vi "Fsweep_SR8XX_2.vi"() -> ()   [LabVIEW 2024]
panel:
  out "Array":dbl[](array[numeric])=[40.99999999999999, 41.74838432440391, 42.51042911458864, 43.28638371880915, 44.07650203674304, 44.88104260256878, 45.70026866956066, 46.53444829622764, 47.38385443402472, 48.248765016665224, 49.129463051063276, 50.02623670993638, 50.93937942609823, 51.86918998847271, 52.815972639860554, 53.78003717649025, 54.761699049386465, 55.76127946758855, 56.779105503253135, 57.81551019867534, 58.87083267526322, 59.94541824450158, 61.039618520941126, 62.153791537250044, 63.28830186136581, 64.44352071578506, 65.61982609903121, 66.81760290933916, 68.03724307059753, 69.27914566059006, 70.5437170415774, 71.83137099326281, 73.14252884818475, 74.47761962958087, 75.83708019176856, 77.22135536308764, 78.6308980914525, 80.0661695925609, 81.5276395008081, 83.01578602295587, 84.53109609460586, 86.07406553952985, 87.64519923190788, 89.24501126152778, 90.87402510200042, 92.53277378204491, 94.22180005990091, 95.94165660092408, 97.6929061584234, 99.47612175779966, 101.29188688404435, 103.14079567266168, 105.02345310407557, 106.94047520158428, 108.89248923292998, 110.88013391554568, 112.90405962555053, 114.96492861055856, 117.06341520637208, 119.20020605763142, 121.37600034249118, 123.59151000139757, 125.84745997004288, 128.14458841657034, 130.48364698311073, 132.8654010317256, 135.2906298948422, 137.76012713025767, 140.27470078079847, 142.8351736387203, 145.44238351493328, 148.09718351314098, 150.80044230898505, 153.55304443428304, 156.35589056645665, 159.2098978232407, 162.11600006277385, 165.07514818916525, 168.08831046363892, 171.15647282135896, 174.28063919403635, 177.46183183842433, 180.70109167081173, 183.9994786076192, 187.35807191221528, 190.77797054806013, 194.26029353829807, 197.80618033191195, 201.41679117656102, 205.09330749822615, 208.83693228778293, 212.64889049463108, 216.53042942751085, 220.4828191626326, 224.50735295925946, 228.60534768287218, 232.7781442360615, 237.02710799728362, 241.353629267624, 245.75912372571858, 250.2450328909765, 254.81282459525804, 259.46399346316485, 264.2000614010933, 269.02257809521853, 273.93312151856446, 278.93329844733324, 284.02474498665686, 289.20912710594536, 294.4881411840093, 299.8635145641304, 305.3370061192634, 310.91040682755784, 316.58554035838205, 322.36426366904453, 328.2484676124084, 334.24007755559677, 340.341054009991, 346.55339327272696, 352.87912807990466, 359.3203282717176, 365.8791014697228, 372.55759376647694, 379.35799042775693, 386.28251660759867, 393.33343807638926, 400.5130619622492, 407.823737505946, 415.26785682958644, 422.847855719344, 430.5662144224702, 438.42545845885314, 446.4281594473945, 454.5769359474659, 462.8744543157258, 471.3234295785769, 479.92662632054976, 488.6868595889001, 497.60699581471715, 506.68995375085, 515.9387054269498, 525.356277121944, 534.9457503542673, 544.7102628901607, 554.6530097703788, 564.7772443556371, 575.086279391144, 585.5834880905614, 596.2723052397499, 607.1562283206671, 618.2388186557745, 629.5237025733345, 641.0145725939827, 652.7151886389541, 664.6293792603626, 676.7610428939417, 689.1141491346505, 701.6927400355609, 714.5009314304542, 727.5429142805647, 740.8229560458996, 754.3454020815899, 768.1146770597366, 782.1352864172023, 796.411817829832, 810.9489427135836, 825.7514177530663, 840.8240864579619, 856.1718807478732, 871.7998225660953, 887.7130255228415, 903.9166965684622, 920.416137697213, 937.2167476821156, 954.3240238414847, 971.7435638377035, 989.4810675088389, 1007.5423387336702, 1025.9332873307803, 1044.659930992305, 1063.7283972529765, 1083.1449254951083, 1102.9158689901853, 1123.0476969777121, 1143.5469967820063, 1164.4204759676343, 1185.6749645341988, 1207.3174171511644, 1229.3549154334992, 1251.7946702588479, 1274.644024126997, 1297.9104535624053, 1321.6015715606015, 1345.725130079225, 1370.2890225745357, 1395.3012865842295, 1420.770106357407, 1446.7038155325192, 1473.1108998642226, 1500.0000000000005]
  in  "data acq time (s)":dbl=2.0
  in  "restart":bool
  in  "stop":bool
  in  "coupled device":enum16{"SRS 8XXX", "Keithley 6221"}(ring)
  in  "base delay (ms)":dbl=2000.0
  in  "test mode":bool
  out "done":u32
  out "delays (ms)":dbl[](array[numeric])=[4439.024390243903, 4395.302276201986, 4352.363927695151, 4310.195294890093, 4268.7825798117565, 4228.112231828511, 4188.170943218251, 4148.945644813986, 4110.423501727488, 4072.5919091495875, 4035.438488225769, 3998.9510820056885, 3963.1177514653054, 3927.9267716003233, 3893.3666275896503, 3859.4260110276505, 3826.093816223921, 3793.359136569407, 3761.2112609676556, 3729.639670330042, 3698.634034133829, 3668.184207041918, 3638.2802255832016, 3608.9123048924207, 3580.0708355084616, 3551.7463802300545, 3523.9296710278295, 3496.6116060117283, 3469.7832464527837, 3443.435813858278, 3417.5606870993415, 3392.1493995900364, 3367.1936365170095, 3342.685232118807, 3318.6161670139577, 3294.978565576961, 3271.7646933613037, 3248.966954568677, 3226.577889563561, 3204.590172432356, 3182.996608586284, 3161.790132407242, 3140.96380493587, 3120.5108116010574, 3100.4244599901485, 3080.698177659125, 3061.3255099820385, 3042.300118038996, 3023.615776542007, 3005.2663717980067, 2987.2458997084013, 2969.5484638044713, 2952.168273317985, 2935.099641286413, 2918.3369826920916, 2901.8748126347614, 2885.707744536847, 2869.8304883809224, 2854.2378489787707, 2838.9247242714628, 2823.8861036599187, 2809.117066365394, 2794.612779819349, 2780.3684980821945, 2766.379560290368, 2752.6413891312604, 2739.149489345473, 2725.899446255926, 2712.8869243233385, 2700.1076657275935, 2687.557488974543, 2675.232287527783, 2663.128028464952, 2651.2407511581287, 2639.566565977868, 2628.101653020485, 2616.8422608581413, 2605.7847053113446, 2594.9253682434514, 2584.2606963767767, 2573.787200129926, 2563.501452475979, 2553.4000878211227, 2543.4798009034093, 2533.7373457112326, 2524.1695344212103, 2514.7732363550926, 2505.5453769553787, 2496.48293677929, 2487.582950510781, 2478.842505990259, 2470.2587432616997, 2461.82885363684, 2453.5500787761516, 2445.4197097862834, 2437.435086333688, 2429.5935957741353, 2421.8926722978285, 2414.3297960898503, 2406.902492505653, 2399.608331261331, 2392.4449256384128, 2385.4099317029, 2378.5010475383115, 2371.716012492475, 2365.05260643782, 2358.508649044931, 2352.081999069123, 2345.7705536498065, 2339.5722476224114, 2333.485052842644, 2327.5069775228635, 2321.6360655803446, 2315.8703959972327, 2310.208082191967, 2304.6472714019756, 2299.1861440774296, 2293.8229132858723, 2288.5558241275194, 2283.383153161035, 2278.303207839608, 2273.3143259571366, 2268.4148751043335, 2263.6032521345915, 2258.8778826394155, 2254.2372204332623, 2249.679747047615, 2245.2039712341216, 2240.808428476652, 2236.4916805120865, 2232.252314859708, 2228.0889443590218, 2224.000206715866, 2219.984764056654, 2216.0413024906106, 2212.1685316798544, 2208.3651844171877, 2204.6300162114517, 2200.9618048803213, 2197.359350150392, 2193.8214732644415, 2190.347016595727, 2186.934843269201, 2183.583836789513, 2180.292900675684, 2177.060958102325, 2173.8869515472916, 2170.769842445651, 2167.7086108498565, 2164.702255096007, 2161.749791476097, 2158.8502539161354, 2156.0026936600393, 2153.2061789591885, 2150.4597947675525, 2147.762642442277, 2145.113839449639, 2142.512519076273, 2139.9578301455767, 2137.4489367391966, 2134.9850179235054, 2132.565267480989, 2130.1888936464406, 2127.85511884789, 2125.563179452175, 2123.312325515071, 2121.1018205359037, 2118.9309412165603, 2116.7989772248175, 2114.7052309619144, 2112.6490173342927, 2110.629663529427, 2108.6465087956735, 2106.698904226067, 2104.786212545992, 2102.90780790466, 2101.0630756703254, 2099.2514122291723, 2097.4722247878076, 2095.72493117929, 2094.008959672643, 2092.3237487857773, 2090.66874710177, 2089.043413088433, 2087.4472149211224, 2085.8796303087165, 2084.3401463227196, 2082.828259229428, 4439.024390243903, 4395.302276201986, 4352.363927695151, 4310.195294890093, 4268.7825798117565, 4228.112231828511, 4439.024390243903, 4395.302276201986, 4352.363927695151, 4310.195294890093, 4268.7825798117565, 4228.112231828511]
  in  "back to initial frequencies":bool=TRUE
  out "delay sum (min)":dbl=15.99183417152745
  in  "index offset":u16=150
  out "freq profile":dbl[][](array[numeric])=[[40.99999999999999, 45.70026866956066, 50.93937942609823], [41.74838432440391, 46.53444829622764, 51.86918998847271], [42.51042911458864, 47.38385443402472, 52.815972639860554], [43.28638371880915, 48.248765016665224, 53.78003717649025], [44.07650203674304, 49.129463051063276, 54.761699049386465], [44.88104260256878, 50.02623670993638, 55.76127946758855], [45.70026866956066, 50.93937942609823, 56.779105503253135], [46.53444829622764, 51.86918998847271, 57.81551019867534], [47.38385443402472, 52.815972639860554, 58.87083267526322], [48.248765016665224, 53.78003717649025, 59.94541824450158], [49.129463051063276, 54.761699049386465, 61.039618520941126], [50.02623670993638, 55.76127946758855, 62.153791537250044], [50.93937942609823, 56.779105503253135, 63.28830186136581], [51.86918998847271, 57.81551019867534, 64.44352071578506], [52.815972639860554, 58.87083267526322, 65.61982609903121], [53.78003717649025, 59.94541824450158, 66.81760290933916], [54.761699049386465, 61.039618520941126, 68.03724307059753], [55.76127946758855, 62.153791537250044, 69.27914566059006], [56.779105503253135, 63.28830186136581, 70.5437170415774], [57.81551019867534, 64.44352071578506, 71.83137099326281], [58.87083267526322, 65.61982609903121, 73.14252884818475], [59.94541824450158, 66.81760290933916, 74.47761962958087], [61.039618520941126, 68.03724307059753, 75.83708019176856], [62.153791537250044, 69.27914566059006, 77.22135536308764], [63.28830186136581, 70.5437170415774, 78.6308980914525], [64.44352071578506, 71.83137099326281, 80.0661695925609], [65.61982609903121, 73.14252884818475, 81.5276395008081], [66.81760290933916, 74.47761962958087, 83.01578602295587], [68.03724307059753, 75.83708019176856, 84.53109609460586], [69.27914566059006, 77.22135536308764, 86.07406553952985], [70.5437170415774, 78.6308980914525, 87.64519923190788], [71.83137099326281, 80.0661695925609, 89.24501126152778], [73.14252884818475, 81.5276395008081, 90.87402510200042], [74.47761962958087, 83.01578602295587, 92.53277378204491], [75.83708019176856, 84.53109609460586, 94.22180005990091], [77.22135536308764, 86.07406553952985, 95.94165660092408], [78.6308980914525, 87.64519923190788, 97.6929061584234], [80.0661695925609, 89.24501126152778, 99.47612175779966], [81.5276395008081, 90.87402510200042, 101.29188688404435], [83.01578602295587, 92.53277378204491, 103.14079567266168], [84.53109609460586, 94.22180005990091, 105.02345310407557], [86.07406553952985, 95.94165660092408, 106.94047520158428], [87.64519923190788, 97.6929061584234, 108.89248923292998], [89.24501126152778, 99.47612175779966, 110.88013391554568], [90.87402510200042, 101.29188688404435, 112.90405962555053], [92.53277378204491, 103.14079567266168, 114.96492861055856], [94.22180005990091, 105.02345310407557, 117.06341520637208], [95.94165660092408, 106.94047520158428, 119.20020605763142], [97.6929061584234, 108.89248923292998, 121.37600034249118], [99.47612175779966, 110.88013391554568, 123.59151000139757], [101.29188688404435, 112.90405962555053, 125.84745997004288], [103.14079567266168, 114.96492861055856, 128.14458841657034], [105.02345310407557, 117.06341520637208, 130.48364698311073], [106.94047520158428, 119.20020605763142, 132.8654010317256], [108.89248923292998, 121.37600034249118, 135.2906298948422], [110.88013391554568, 123.59151000139757, 137.76012713025767], [112.90405962555053, 125.84745997004288, 140.27470078079847], [114.96492861055856, 128.14458841657034, 142.8351736387203], [117.06341520637208, 130.48364698311073, 145.44238351493328], [119.20020605763142, 132.8654010317256, 148.09718351314098], [121.37600034249118, 135.2906298948422, 150.80044230898505], [123.59151000139757, 137.76012713025767, 153.55304443428304], [125.84745997004288, 140.27470078079847, 156.35589056645665], [128.14458841657034, 142.8351736387203, 159.2098978232407], [130.48364698311073, 145.44238351493328, 162.11600006277385], [132.8654010317256, 148.09718351314098, 165.07514818916525], [135.2906298948422, 150.80044230898505, 168.08831046363892], [137.76012713025767, 153.55304443428304, 171.15647282135896], [140.27470078079847, 156.35589056645665, 174.28063919403635], [142.8351736387203, 159.2098978232407, 177.46183183842433], [145.44238351493328, 162.11600006277385, 180.70109167081173], [148.09718351314098, 165.07514818916525, 183.9994786076192], [150.80044230898505, 168.08831046363892, 187.35807191221528], [153.55304443428304, 171.15647282135896, 190.77797054806013], [156.35589056645665, 174.28063919403635, 194.26029353829807], [159.2098978232407, 177.46183183842433, 197.80618033191195], [162.11600006277385, 180.70109167081173, 201.41679117656102], [165.07514818916525, 183.9994786076192, 205.09330749822615], [168.08831046363892, 187.35807191221528, 208.83693228778293], [171.15647282135896, 190.77797054806013, 212.64889049463108], [174.28063919403635, 194.26029353829807, 216.53042942751085], [177.46183183842433, 197.80618033191195, 220.4828191626326], [180.70109167081173, 201.41679117656102, 224.50735295925946], [183.9994786076192, 205.09330749822615, 228.60534768287218], [187.35807191221528, 208.83693228778293, 232.7781442360615], [190.77797054806013, 212.64889049463108, 237.02710799728362], [194.26029353829807, 216.53042942751085, 241.353629267624], [197.80618033191195, 220.4828191626326, 245.75912372571858], [201.41679117656102, 224.50735295925946, 250.2450328909765], [205.09330749822615, 228.60534768287218, 254.81282459525804], [208.83693228778293, 232.7781442360615, 259.46399346316485], [212.64889049463108, 237.02710799728362, 264.2000614010933], [216.53042942751085, 241.353629267624, 269.02257809521853], [220.4828191626326, 245.75912372571858, 273.93312151856446], [224.50735295925946, 250.2450328909765, 278.93329844733324], [228.60534768287218, 254.81282459525804, 284.02474498665686], [232.7781442360615, 259.46399346316485, 289.20912710594536], [237.02710799728362, 264.2000614010933, 294.4881411840093], [241.353629267624, 269.02257809521853, 299.8635145641304], [245.75912372571858, 273.93312151856446, 305.3370061192634], [250.2450328909765, 278.93329844733324, 310.91040682755784], [254.81282459525804, 284.02474498665686, 316.58554035838205], [259.46399346316485, 289.20912710594536, 322.36426366904453], [264.2000614010933, 294.4881411840093, 328.2484676124084], [269.02257809521853, 299.8635145641304, 334.24007755559677], [273.93312151856446, 305.3370061192634, 340.341054009991], [278.93329844733324, 310.91040682755784, 346.55339327272696], [284.02474498665686, 316.58554035838205, 352.87912807990466], [289.20912710594536, 322.36426366904453, 359.3203282717176], [294.4881411840093, 328.2484676124084, 365.8791014697228], [299.8635145641304, 334.24007755559677, 372.55759376647694], [305.3370061192634, 340.341054009991, 379.35799042775693], [310.91040682755784, 346.55339327272696, 386.28251660759867], [316.58554035838205, 352.87912807990466, 393.33343807638926], [322.36426366904453, 359.3203282717176, 400.5130619622492], [328.2484676124084, 365.8791014697228, 407.823737505946], [334.24007755559677, 372.55759376647694, 415.26785682958644], [340.341054009991, 379.35799042775693, 422.847855719344], [346.55339327272696, 386.28251660759867, 430.5662144224702], [352.87912807990466, 393.33343807638926, 438.42545845885314], [359.3203282717176, 400.5130619622492, 446.4281594473945], [365.8791014697228, 407.823737505946, 454.5769359474659], [372.55759376647694, 415.26785682958644, 462.8744543157258], [379.35799042775693, 422.847855719344, 471.3234295785769], [386.28251660759867, 430.5662144224702, 479.92662632054976], [393.33343807638926, 438.42545845885314, 488.6868595889001], [400.5130619622492, 446.4281594473945, 497.60699581471715], [407.823737505946, 454.5769359474659, 506.68995375085], [415.26785682958644, 462.8744543157258, 515.9387054269498], [422.847855719344, 471.3234295785769, 525.356277121944], [430.5662144224702, 479.92662632054976, 534.9457503542673], [438.42545845885314, 488.6868595889001, 544.7102628901607], [446.4281594473945, 497.60699581471715, 554.6530097703788], [454.5769359474659, 506.68995375085, 564.7772443556371], [462.8744543157258, 515.9387054269498, 575.086279391144], [471.3234295785769, 525.356277121944, 585.5834880905614], [479.92662632054976, 534.9457503542673, 596.2723052397499], [488.6868595889001, 544.7102628901607, 607.1562283206671], [497.60699581471715, 554.6530097703788, 618.2388186557745], [506.68995375085, 564.7772443556371, 629.5237025733345], [515.9387054269498, 575.086279391144, 641.0145725939827], [525.356277121944, 585.5834880905614, 652.7151886389541], [534.9457503542673, 596.2723052397499, 664.6293792603626], [544.7102628901607, 607.1562283206671, 676.7610428939417], [554.6530097703788, 618.2388186557745, 689.1141491346505], [564.7772443556371, 629.5237025733345, 701.6927400355609], [575.086279391144, 641.0145725939827, 714.5009314304542], [585.5834880905614, 652.7151886389541, 727.5429142805647], [596.2723052397499, 664.6293792603626, 740.8229560458996], [607.1562283206671, 676.7610428939417, 754.3454020815899], [618.2388186557745, 689.1141491346505, 768.1146770597366], [629.5237025733345, 701.6927400355609, 782.1352864172023], [641.0145725939827, 714.5009314304542, 796.411817829832], [652.7151886389541, 727.5429142805647, 810.9489427135836], [664.6293792603626, 740.8229560458996, 825.7514177530663], [676.7610428939417, 754.3454020815899, 840.8240864579619], [689.1141491346505, 768.1146770597366, 856.1718807478732], [701.6927400355609, 782.1352864172023, 871.7998225660953], [714.5009314304542, 796.411817829832, 887.7130255228415], [727.5429142805647, 810.9489427135836, 903.9166965684622], [740.8229560458996, 825.7514177530663, 920.416137697213], [754.3454020815899, 840.8240864579619, 937.2167476821156], [768.1146770597366, 856.1718807478732, 954.3240238414847], [782.1352864172023, 871.7998225660953, 971.7435638377035], [796.411817829832, 887.7130255228415, 989.4810675088389], [810.9489427135836, 903.9166965684622, 1007.5423387336702], [825.7514177530663, 920.416137697213, 1025.9332873307803], [840.8240864579619, 937.2167476821156, 1044.659930992305], [856.1718807478732, 954.3240238414847, 1063.7283972529765], [871.7998225660953, 971.7435638377035, 1083.1449254951083], [887.7130255228415, 989.4810675088389, 1102.9158689901853], [903.9166965684622, 1007.5423387336702, 1123.0476969777121], [920.416137697213, 1025.9332873307803, 1143.5469967820063], [937.2167476821156, 1044.659930992305, 1164.4204759676343], [954.3240238414847, 1063.7283972529765, 1185.6749645341988], [971.7435638377035, 1083.1449254951083, 1207.3174171511644], [989.4810675088389, 1102.9158689901853, 1229.3549154334992], [1007.5423387336702, 1123.0476969777121, 1251.7946702588479], [1025.9332873307803, 1143.5469967820063, 1274.644024126997], [1044.659930992305, 1164.4204759676343, 1297.9104535624053], [1063.7283972529765, 1185.6749645341988, 1321.6015715606015], [1083.1449254951083, 1207.3174171511644, 1345.725130079225], [1102.9158689901853, 1229.3549154334992, 1370.2890225745357], [1123.0476969777121, 1251.7946702588479, 1395.3012865842295], [1143.5469967820063, 1274.644024126997, 1420.770106357407], [1164.4204759676343, 1297.9104535624053, 1446.7038155325192], [1185.6749645341988, 1321.6015715606015, 1473.1108998642226], [1207.3174171511644, 1345.725130079225, 1500.0000000000005], [1229.3549154334992, 1370.2890225745357, 40.99999999999999], [1251.7946702588479, 1395.3012865842295, 41.74838432440391], [1274.644024126997, 1420.770106357407, 42.51042911458864], [1297.9104535624053, 1446.7038155325192, 43.28638371880915], [1321.6015715606015, 1473.1108998642226, 44.07650203674304], [1345.725130079225, 1500.0000000000005, 44.88104260256878], [1370.2890225745357, 40.99999999999999, 45.70026866956066], [1395.3012865842295, 41.74838432440391, 46.53444829622764], [1420.770106357407, 42.51042911458864, 47.38385443402472], [1446.7038155325192, 43.28638371880915, 48.248765016665224], [1473.1108998642226, 44.07650203674304, 49.129463051063276], [1500.0000000000005, 44.88104260256878, 50.02623670993638]]
  out "freqs":dbl[](array[numeric])=[44.88104260256878, 676.7610428939417, 273.93312151856446]
  out "delay (ms)":dbl=4228.112231828511
  out "elapsed time (min)":dbl=0.7130166666666666
  in  "sweep mode":T1(ring)=enum."log"
  in  "size":u32=200
  in  "final":dbl=1500.0
  in  "initial":dbl=41.0
  in  "Device address":refnum<visa-resource-name>[](array[refnum])=["GPIB0::1::INSTR", "GPIB0::4::INSTR", "GPIB0::7::INSTR"]
  # "Test the frequency profile and the estimated measurement time (delay sum (min)) with the 'test mode on'\nTurn the test mode off for the real measurement."
  # "Start data acquistion  and frequency sweeps.\nStop the data acqusition when the sweep is done.\nRepeat when 'restart' switch is ON.\nVISA resource is reused."
  # "this delay time is added to the frequency dependent delay time"
  # "(1) For multiple lockins, the same freq profile is used but\nbut the starting frequency is offset to prevent crosstalking.\n(2) Ignored for a single lockin. \n* Check the context help"
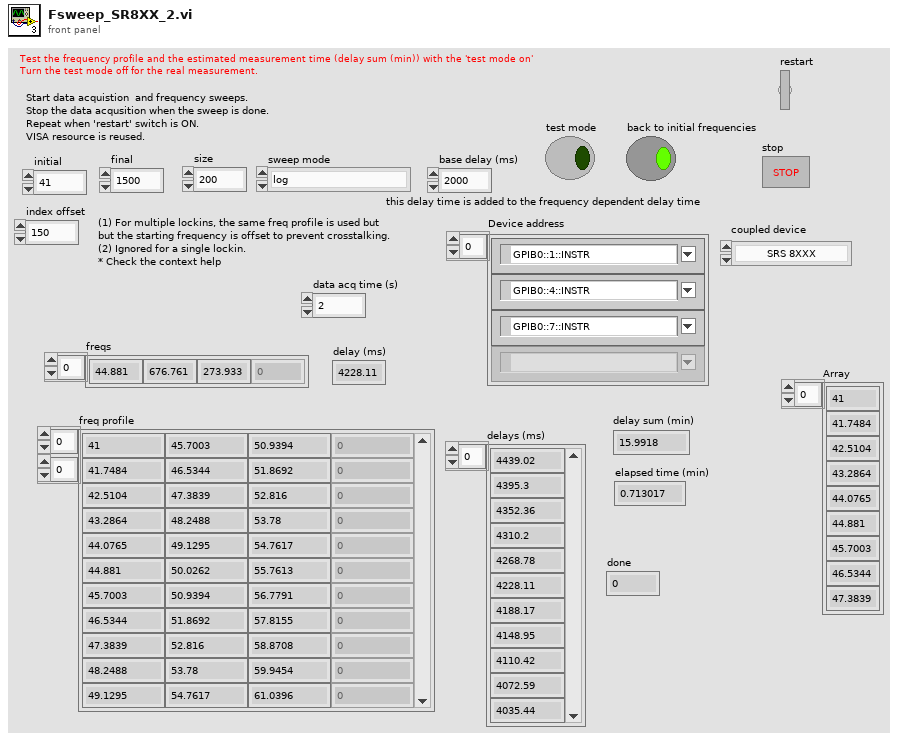
[diagram p1: front panel]
types:
  T1 = enum16{"linear", "inverse", "log", "inverse log"}
  T2 = enum32{"New", "Stop", "Trigger", "Delta Trigger", "Run", "Pause", "comments", "Started?"}
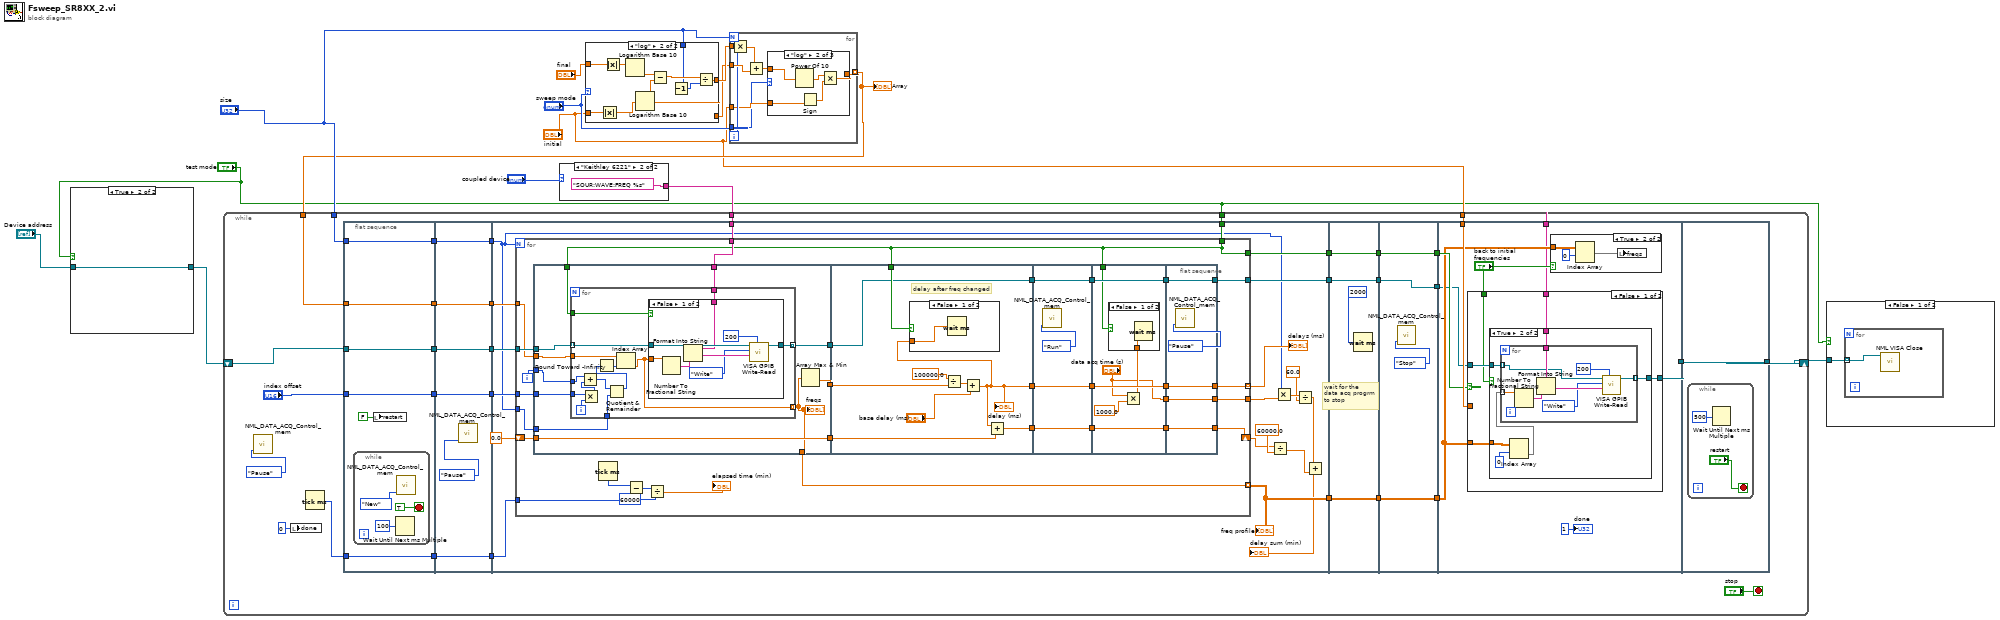
[diagram p0: block diagram]
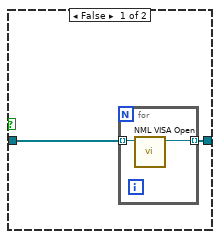
[diagram p3: hidden frame]
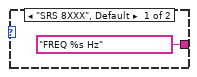
[diagram p10: hidden frame]
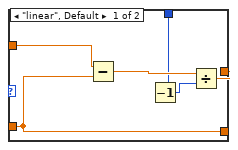
[diagram p11: hidden frame]
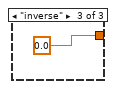
[diagram p13: hidden frame]
diagram:
  n1 = case shown="True" "test mode" {
    tunnel: [w15 w18] -> w4
    tunnel: "Device address" -> [w14 w18]
    frame False {
      n2 = for {
        tunnel: w14 -> [w17] mode=indexing
        tunnel: [w16] -> w15 mode=indexing
        n3 = call "NML VISA Open.vi"("VISA resource name"=w17) -> ("VISA resource name out"=w16:refnum<visa-resource-name>)  [unwired: 9 in, 1 out]
      }
    }
    frame True {
    }
  }
  n4 = case shown="\"Keithley 6221\"" "coupled device" {
    tunnel: ["FREQ %s Hz" ("format string") "SOUR:WAVE:FREQ %s" ("format string")] -> w5
    frame "SRS 8XXX", Default {
    }
    frame "Keithley 6221" {
    }
  }
  n5 = case shown="\"log\"" "sweep mode" {
    tunnel: "final" -> [w26 w27]
    tunnel: "initial" -> [w21 w32]
    tunnel: "size" -> [w24 w35]
    tunnel: [w23 w34] -> w13
    tunnel: [w21 w28] -> w12
    frame "linear", Default {
      n6 = Subtract(x=w26, y=w21) -> (x-y=w25:dbl)
      n7 = Decrement(x=w24) -> (x-1=w22:u32)
      n8 = Divide(x=w25, y=w22) -> (x/y=w23:dbl)
    }
    frame "log" {
      n9 = Absolute Value(x=w32) -> (abs(x)=w29:dbl)
      n10 = Absolute Value(x=w27) -> (abs(x)=w30:dbl)
      n11 = Logarithm Base 10(1:w30) -> (0:w31:dbl)
      n12 = Logarithm Base 10(1:w29) -> (0:w28:dbl)
      n13 = Subtract(x=w31, y=w28) -> (x-y=w36:dbl)
      n14 = Decrement(x=w35) -> (x-1=w33:u32)
      n15 = Divide(x=w36, y=w33) -> (x/y=w34:dbl)
    }
  }
  n16 = for {
    N: "size" -> [_]
    tunnel: w13 -> [w42]
    tunnel: [w44] -> w8 mode=indexing
    tunnel: "sweep mode" -> [w37]
    tunnel: w12 -> [w40]
    tunnel: "initial" -> [w38]
    i -> [w39]
    n17 = Multiply(x=w42, y=w39) -> (x*y=w41:dbl)
    n18 = Add(x=w41, y=w40) -> (x+y=w43:dbl)
    n19 = case shown="\"log\"" w37 {
      tunnel: [w45 w48 0.0] -> w44
      tunnel: w43 -> [w45 w50 _]
      tunnel: w38 -> [_ w47 _]
      frame "linear", Default {
      }
      frame "log" {
        n20 = Power Of 10(x=w50) -> (10^x=w49:dbl)
        n21 = Sign(1:w47) -> (0:w46:dbl)
        n22 = Multiply(x=w49, y=w46) -> (x*y=w48:dbl)
      }
      frame "inverse" {
      }
    }
  }
  "Array" <- w8
  n23 = while {
    tunnel: "size" -> [w54]
    tunnel: w8 -> [w61]
    tunnel: "initial" -> [w60]
    tunnel: w5 -> [w59]
    shift-right: [w57] -> w3
    shift-left: w4 -> [w58]
    tunnel: "test mode" -> [w52]
    stop <- "stop" stop-if-true
    n24 = call "NML_DATA_ACQ_Control_mem.vi"("Enum"=T2."Pause") -> ()  [unwired: 4 in, 1 out]
    n25 = local write "done"(u32 0 ("done")) -> ()
    n26 = Tick Count (ms)() -> (millisecond timer value=w64:u32)
    n27 = flat-sequence {
      tunnel: "index offset" -> [w85]
      tunnel: w58 -> [w86]
      tunnel: w54 -> [w87]
      tunnel: w64 -> [w88]
      tunnel: w61 -> [w89]
      tunnel: [w89] -> w83
      tunnel: [w88] -> w82
      tunnel: [w87] -> w81
      tunnel: [w86] -> w80
      tunnel: [w85] -> w79
      tunnel: w83 -> [w98]
      tunnel: [w98] -> w78
      tunnel: w82 -> [w97]
      tunnel: [w97] -> w77
      tunnel: w81 -> [w96]
      tunnel: [w96] -> w76
      tunnel: w80 -> [w95]
      tunnel: [w95] -> w75
      tunnel: w79 -> [w94]
      tunnel: [w94] -> w74
      tunnel: [w117] -> w73
      tunnel: [w110] -> w72
      tunnel: w59 -> [w108]
      tunnel: [w107] -> w71
      tunnel: w78 -> [w118]
      tunnel: w77 -> [w116]
      tunnel: w76 -> [w104]
      tunnel: w75 -> [w111]
      tunnel: w74 -> [w115]
      tunnel: w52 -> [w106]
      tunnel: w73 -> [w214]
      tunnel: [w214] -> w70
      tunnel: w72 -> [w213]
      tunnel: [w213] -> w69
      tunnel: w71 -> [w212]
      tunnel: [w212] -> w68
      tunnel: w70 -> [w218]
      tunnel: [w218] -> w67
      tunnel: w69 -> [w217]
      tunnel: [w217] -> w66
      tunnel: [w216] -> w65
      tunnel: w68 -> [w216]
      tunnel: w67 -> [w225]
      tunnel: w60 -> [w226]
      tunnel: w66 -> [w222]
      tunnel: w59 -> [w221]
      tunnel: w65 -> [w219]
      tunnel: [w220] -> w53
      tunnel: [w251] -> w57
      tunnel: w53 -> [w251]
      frame #0 {
        n28 = while {
          stop <- TRUE stop-if-true
          n29 = Wait Until Next ms Multiple(millisecond multiple=u32 100) -> ()  [unwired: 1 out]
          n30 = call "NML_DATA_ACQ_Control_mem.vi"("Enum"=T2."New") -> ()  [unwired: 4 in, 1 out]
        }
        n31 = local write "restart"(FALSE ("restart")) -> ()
      }
      frame #1 {
        n32 = call "NML_DATA_ACQ_Control_mem.vi"("Enum"=T2."Pause") -> ()  [unwired: 4 in, 1 out]
      }
      frame #2 {
        n33 = for {
          N: w104 -> [_]
          tunnel: w118 -> [w135]
          tunnel: [w120] -> w117
          tunnel: w116 -> [w148]
          tunnel: w111 -> [w144]
          tunnel: w115 -> [w142]
          tunnel: w104 -> [w141]
          tunnel: [w136] -> w110 mode=indexing
          tunnel: [w119] -> w109 mode=indexing
          shift-right: [w139] -> w112
          shift-left: 0.0 -> [w137]
          tunnel: w108 -> [w134]
          tunnel: [w133] -> w107
          tunnel: w106 -> [w120]
          tunnel: [w121] -> w105
          i -> [w143]
          n34 = flat-sequence {
            tunnel: w135 -> [w158]
            tunnel: w120 -> [w160]
            tunnel: w144 -> [w159]
            tunnel: w143 -> [w157]
            tunnel: w142 -> [w156]
            tunnel: w141 -> [w155]
            tunnel: [w153] -> w140
            tunnel: [w152] -> w136
            tunnel: [w154] -> w138
            tunnel: w137 -> [w154]
            tunnel: w134 -> [w151]
            tunnel: [w150] -> w132
            tunnel: w140 -> [w191]
            tunnel: w120 -> [w189]
            tunnel: w138 -> [w186]
            tunnel: w132 -> [w184]
            tunnel: [w188] -> w131
            tunnel: [w187] -> w130
            tunnel: [w184] -> w129
            tunnel: w131 -> [w197]
            tunnel: w130 -> [w196]
            tunnel: w129 -> [w195]
            tunnel: [w197] -> w128
            tunnel: [w196] -> w127
            tunnel: [w195] -> w126
            tunnel: w128 -> [w204]
            tunnel: w127 -> [w203]
            tunnel: w126 -> [w202]
            tunnel: [w204] -> w125
            tunnel: [w203] -> w124
            tunnel: [w202] -> w123
            tunnel: ["data acq time (s)"] -> w122
            tunnel: w120 -> [w199]
            tunnel: [w208] -> w133
            tunnel: [w209] -> w139
            tunnel: [w210] -> w119
            tunnel: w125 -> [w210]
            tunnel: w124 -> [w209]
            tunnel: w123 -> [w208]
            tunnel: w122 -> [w206]
            tunnel: [w206] -> w121
            frame #0 {
              n35 = for {
                tunnel: w160 -> [w174]
                tunnel: w159 -> [w173] mode=indexing
                tunnel: w158 -> [w168]
                tunnel: w157 -> [w171]
                tunnel: w156 -> [w170]
                tunnel: [w165] -> w152 mode=indexing
                tunnel: w155 -> [w166]
                tunnel: w151 -> [w162]
                tunnel: [w161] -> w150 mode=indexing
                i -> [w172]
                n36 = Multiply(x=w170, y=w172) -> (x*y=w169:i32)
                n37 = Add(x=w171, y=w169) -> (x+y=w167:i32)
                n38 = Quotient & Remainder(x=w167, y=w166) -> (x-y*floor(x/y)=w164:u32)  [unwired: 1 out]
                n39 = Round Toward -Infinity(1:w164) -> (0:w163:u32)
                n40 = Index Array(array=w168, index=w163) -> (element=w165:dbl)
                n41 = case shown="False" w174 {
                  tunnel: w173 -> [w178 w183]
                  tunnel: w165 -> [w177 _]
                  tunnel: w162 -> [w176 _]
                  tunnel: [w175 w183] -> w161
                  frame False {
                    n42 = Number To Fractional String(number=w177) -> (F-format string=w181:string)  [unwired: 3 in]
                    n43 = Format Into String(format string=w176, w181) -> (resulting string=w182:string)  [unwired: 2 in, 1 out]
                    n44 = call "VISA GPIB Write-Read.vi"("Wait (ms)"=u32 200 ("wait (mS)"), "Command"=w182, "Action"=enum16{"Write", "Read", "Write & Read"}."Write", "VISA resource name"=w178) -> ("dup VISA Session"=w175:refnum<visa-resource-name>)  [unwired: 4 in, 3 out]
                  }
                  frame True {
                  }
                }
              }
              "freqs" <- w152
              n45 = Array Max & Min(array=w152) -> (min value=w153:dbl)  [unwired: 3 out]
            }
            frame #1 {
              # "delay after freq changed"
              n46 = Divide(x=100000.0, y=w191) -> (x/y=w192:dbl)
              n47 = Add(x=w192, y="base delay (ms)") -> (x+y=w188:dbl)
              "delay (ms)" <- w188
              n48 = case shown="False" w189 {
                tunnel: w188 -> [w193 _]
                frame False {
                  n49 = Wait (ms)(milliseconds to wait=w193) -> ()  [unwired: 1 out]
                }
                frame True {
                }
              }
              n50 = Add(x=w188, y=w186) -> (x+y=w187:dbl)
            }
            frame #2 {
              n51 = call "NML_DATA_ACQ_Control_mem.vi"("Enum"=T2."Run") -> ()  [unwired: 4 in, 1 out]
            }
            frame #3 {
              n52 = Multiply(x="data acq time (s)", y=1000.0) -> (x*y=w200:dbl)
              n53 = case shown="False" w199 {
                tunnel: w200 -> [w205 _]
                frame False {
                  n54 = Wait (ms)(milliseconds to wait=w205) -> ()  [unwired: 1 out]
                }
                frame True {
                }
              }
            }
            frame #4 {
              n55 = call "NML_DATA_ACQ_Control_mem.vi"("Enum"=T2."Pause") -> ()  [unwired: 4 in, 1 out]
            }
          }
          n56 = Tick Count (ms)() -> (millisecond timer value=w149:u32)
          n57 = Subtract(x=w149, y=w148) -> (x-y=w147:u32)
          n58 = Divide(x=w147, y=u32 60000) -> (x/y=→"elapsed time (min)":dbl)
        }
        "freq profile" <- w110
        "delays (ms)" <- w109
        n59 = Divide(x=w112, y=60000.0) -> (x/y=w100:dbl)
        n60 = Multiply(x=w104, y=w105) -> (x*y=w103:dbl)
        n61 = Divide(x=w103, y=60.0) -> (x/y=w101:dbl)
        n62 = Add(x=w101, y=w100) -> (x+y=→"delay sum (min)":dbl)
      }
      frame #3 {
        # "wait for the\ndata acq progrm\nto stop"
        n63 = Wait (ms)(milliseconds to wait=u32 2000) -> ()  [unwired: 1 out]
      }
      frame #4 {
        n64 = call "NML_DATA_ACQ_Control_mem.vi"("Enum"=T2."Stop") -> ()  [unwired: 4 in, 1 out]
      }
      frame #5 {
        n65 = case shown="False" w225 {
          tunnel: w226 -> [_ _]
          tunnel: w219 -> [w234 w250]
          tunnel: w222 -> [w233 _]
          tunnel: "back to initial frequencies" -> [w232 _]
          tunnel: w221 -> [w231 _]
          tunnel: [w230 w250] -> w220
          frame False {
            n66 = case shown="True" w232 {
              tunnel: w234 -> [w235 w241]
              tunnel: w233 -> [_ w240]
              tunnel: w231 -> [_ w237]
              tunnel: [w235 w236] -> w230
              frame False {
              }
              frame True {
                n67 = Index Array(array=w240, index (row)=0) -> (element=w238:dbl[])  [unwired: 1 in]
                n68 = for {
                  tunnel: w241 -> [w242] mode=indexing
                  tunnel: w238 -> [w245] mode=indexing
                  tunnel: w237 -> [w244]
                  tunnel: [w243] -> w236 mode=indexing
                  n69 = Number To Fractional String(number=w245) -> (F-format string=w248:string)  [unwired: 3 in]
                  n70 = Format Into String(format string=w244, w248) -> (resulting string=w249:string)  [unwired: 2 in, 1 out]
                  n71 = call "VISA GPIB Write-Read.vi"("Wait (ms)"=u32 200 ("wait (mS)"), "Command"=w249, "Action"=enum16{"Write", "Read", "Write & Read"}."Write", "VISA resource name"=w242) -> ("dup VISA Session"=w243:refnum<visa-resource-name>)  [unwired: 4 in, 3 out]
                }
              }
            }
          }
          frame True {
          }
        }
        n72 = case shown="True" "back to initial frequencies" {
          tunnel: w222 -> [_ w229]
          frame False {
          }
          frame True {
            n73 = Index Array(array=w229, index (row)=0) -> (element=w227:dbl[])  [unwired: 1 in]
            n74 = local write "freqs"(w227) -> ()
          }
        }
        "done" <- u32 1 ("done")
      }
      frame #6 {
        n75 = while {
          stop <- "restart" stop-if-true
          n76 = Wait Until Next ms Multiple(millisecond multiple=u32 500) -> ()  [unwired: 1 out]
        }
      }
    }
  }
  n77 = case shown="False" "test mode" {
    tunnel: w3 -> [w254 _]
    frame False {
      n78 = for {
        tunnel: w254 -> [w255] mode=indexing
        n79 = call "NML VISA Close.vi"("VISA resource name"=w255) -> ()  [unwired: 10 in, 1 out]
      }
    }
    frame True {
    }
  }
